vi "Get LV Color.vi"(8 "error in (no error)":errorcluster, 11 "Graphics Object.lvclass in":refnum<class "Graphics Object.lvclass">) -> (0 "error out":errorcluster, 2 "Color":u32(colorbox), 3 "Graphics Object.lvclass out":refnum<class "Graphics Object.lvclass">)   [LabVIEW 2020, in "Graphics Object.lvclass"]
doc: "Method for getting the LabVIEW color value corresponding the graphics object color."
uses:
  Graphics Object.lvclass
  Color/Color.lvclass
panel:
  # "expressionflow.com"
  # "Copyright (c) 2008 Tomi Maila. All rights reserved."
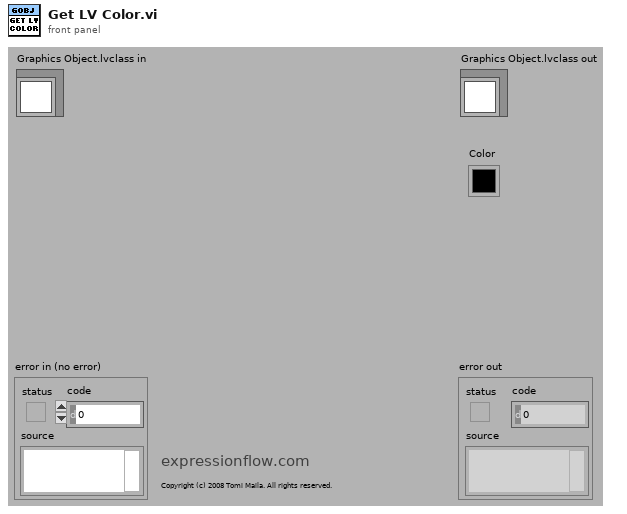
[diagram p1: front panel]
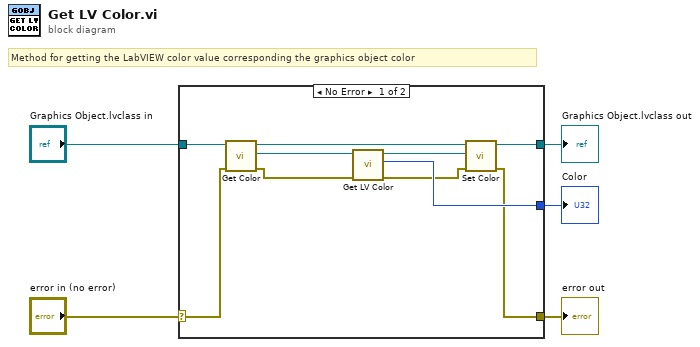
[diagram p0: block diagram]
diagram:
  # "Method for getting the LabVIEW color value corresponding the graphics object color"
  n1 = case shown="No Error" "error in (no error)" {
    selector: "error in (no error)" -> [w13 w16]
    tunnel: [w6 w16] -> w4
    tunnel: [w10 w17] -> w2
    tunnel: "Graphics Object.lvclass in" -> [w14 w17]
    tunnel: [w15 _] -> w1
    frame No Error {
      n2 = call-dynamic "Get Color.vi"("error in (no error)"=w13, "Geometric Object.lvclass in"=w14) -> ("error out"=w12:errorcluster, "Color.lvclass"=w11:refnum<class "Color.lvclass">, "Geometric Object.lvclass out"=w9:refnum<class "Graphics Object.lvclass">)  [unwired: 7 in]
      n3 = call-dynamic "Get LV Color.vi"("error in (no error)"=w12, "Color in"=w11) -> ("error out"=w7:errorcluster, "Color"=w15:u32, "Color out"=w8:refnum<class "Color.lvclass">)  [unwired: 7 in]
      n4 = call-dynamic "Set Color.vi"("error in (no error)"=w7, "Color (RGB black)"=w8, "Geometric Object.lvclass in"=w9) -> ("error out"=w6:errorcluster, "Geometric Object.lvclass out"=w10:refnum<class "Graphics Object.lvclass">)  [unwired: 7 in]
    }
    frame Error {
    }
  }
  "error out" <- w4
  "Graphics Object.lvclass out" <- w2
  "Color" <- w1
